vi "Write Timestamp.vi"(8 "error in (no error)":errorcluster, 10 "Timestamp":timestamp, 11 "LogRecord in":refnum<class "LogRecord.lvclass">) -> (0 "error out":errorcluster, 3 "LogRecord out":refnum<class "LogRecord.lvclass">)   [LabVIEW 2016, in "hse-logger.lvlib" / "LogRecord.lvclass"]
uses:
  LogRecord.lvclass
  LogRecord.lvclass/LogRecord.ctl
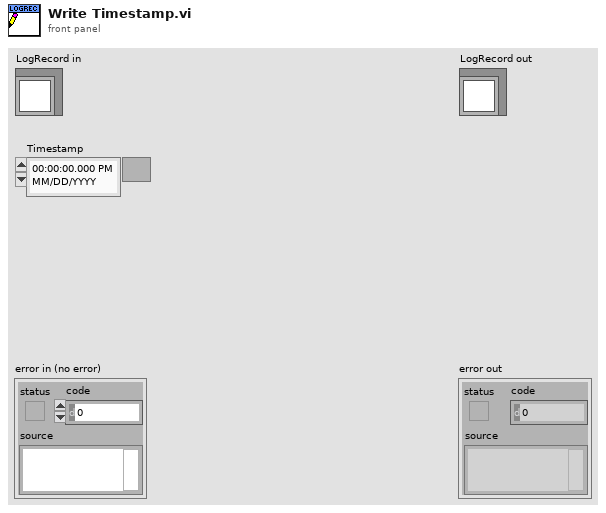
[diagram p1: front panel]
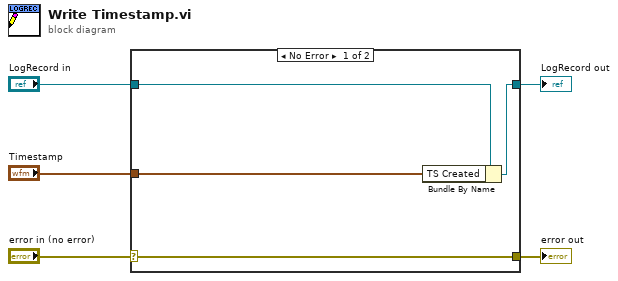
[diagram p0: block diagram]
diagram:
  n1 = case shown="No Error" "error in (no error)" {
    selector: "error in (no error)" -> [w9 w10]
    tunnel: [w9 w10] -> w4
    tunnel: [w7 w11] -> w2
    tunnel: "LogRecord in" -> [w8 w11]
    tunnel: "Timestamp" -> [w6 _]
    frame No Error {
      n2 = Bundle By Name(cluster=w8, "TS Created"=w6) -> (w7:refnum<class "LogRecord.lvclass">)
    }
    frame Error {
    }
  }
  "error out" <- w4
  "LogRecord out" <- w2
